vi "Playback Frame Crop Utility.vi"(8 "error in (no error)":errorcluster, 11 "Frame Grabber Data in":T2={"Camera Session"="", "Frame"=refnum, "AVI Refnum"=refnum, "Codecs"=[], "Frame number"=0, "Tracking File Refnum"=refnum, "Tick Count"=0, "Probe Object"=refnum, "Playback Probe Data"=[], "Rigid Body"={"Position"={"x (mm)"=0.0, "y (mm)"=0.0, "z (mm)"=0.0}, "Orientation"={"Pitch (rad)"=0.0, "Yaw (rad)"=0.0, "Roll (rad)"=0.0}, "Quaternion"={"qx"=0.0, "qy"=0.0, "qz"=0.0, "qw"=0.0}, "Tracked?"=FALSE}, "Total no frames playback"=0, "Video FPS"=0.0, "Camera connected?"=FALSE, "Scene"=refnum, "Cropped Frame"=refnum, "Tracker FPS"=0.0, "Crop ROI"=[], "Presentation Values"=[], "Elapsed time (ms)"=0, "Camera frames playback"=0, "Refnums"={"Live Refnum"=refnum, "Record Refnum"=refnum, "Playback Refnum"=refnum, "Frame Slider Refnum"=refnum, "Pause Refnum"=refnum, "Home Refnum"=refnum, "Set Crop Refnum"=refnum, "Clear Crop Refnum"=refnum, "stop refnum"=refnum, "Playback Rate Refnum"=refnum, "Presentation Refnum"=refnum, "Crop Time Frame Slider Refnum"=refnum, "Cancel Save Refnum"=refnum, "Reverse Playback Refnum"=refnum, "Recording Settings Refnum"=refnum, "Continuous Playback Refnum"=refnum, "Annotation Refnum"=refnum, "Export All Refnum"=refnum, "Export List Refnum"=refnum, "Fill List Refnum"=refnum, "Save Crop Refnum"=refnum, "Skip Forward Refnum"=refnum, "Skip Backward Refnum"=refnum, "Single Annotation Refnum"=refnum, "Load Refnum"=refnum, "Set Start Refnum"=refnum, "Set End Refnum"=refnum, "Add to List Refnum"=refnum, "List of Annotations Refnum"=refnum, "Camera Frame Refnum"=refnum}, "Dimensions"={"Probe Dimensions"={"Probe Width"=0.0, "Probe Depth"=1.0, "Probe Height"=0.0}, "Room Dimensions"={"Room Width"=0.0, "Room Depth"=0.0, "Room Height"=0.0}}, "Playback Data As Strings"=[], "Cropped Tracking File Refnum"=refnum, "Cropped AVI Refnum"=refnum, "Header"=[], "Total euclidian distance"=0.0, "Annotation File Path"=path "", "Playback File Path"=path "", "Size per frame"=0.0, "Ground Truth File Refnum"=refnum, "Annotation Array"=[], "Annotation TIFFs Folder"=path "", "overwriting open file?"=FALSE}) -> (0 "error out":errorcluster, 1 "Continue playback?":bool, 2 "Image":T1, 3 "Frame Grabber Data out":T2={"Camera Session"="", "Frame"=refnum, "AVI Refnum"=refnum, "Codecs"=[], "Frame number"=0, "Tracking File Refnum"=refnum, "Tick Count"=0, "Probe Object"=refnum, "Playback Probe Data"=[], "Rigid Body"={"Position"={"x (mm)"=0.0, "y (mm)"=0.0, "z (mm)"=0.0}, "Orientation"={"Pitch (rad)"=0.0, "Yaw (rad)"=0.0, "Roll (rad)"=0.0}, "Quaternion"={"qx"=0.0, "qy"=0.0, "qz"=0.0, "qw"=0.0}, "Tracked?"=FALSE}, "Total no frames playback"=0, "Video FPS"=0.0, "Camera connected?"=FALSE, "Scene"=refnum, "Cropped Frame"=refnum, "Tracker FPS"=0.0, "Crop ROI"=[], "Presentation Values"=[], "Elapsed time (ms)"=0, "Camera frames playback"=0, "Refnums"={"Live Refnum"=refnum, "Record Refnum"=refnum, "Playback Refnum"=refnum, "Frame Slider Refnum"=refnum, "Pause Refnum"=refnum, "Home Refnum"=refnum, "Set Crop Refnum"=refnum, "Clear Crop Refnum"=refnum, "stop refnum"=refnum, "Playback Rate Refnum"=refnum, "Presentation Refnum"=refnum, "Crop Time Frame Slider Refnum"=refnum, "Cancel Save Refnum"=refnum, "Reverse Playback Refnum"=refnum, "Recording Settings Refnum"=refnum, "Continuous Playback Refnum"=refnum, "Annotation Refnum"=refnum, "Export All Refnum"=refnum, "Export List Refnum"=refnum, "Fill List Refnum"=refnum, "Save Crop Refnum"=refnum, "Skip Forward Refnum"=refnum, "Skip Backward Refnum"=refnum, "Single Annotation Refnum"=refnum, "Load Refnum"=refnum, "Set Start Refnum"=refnum, "Set End Refnum"=refnum, "Add to List Refnum"=refnum, "List of Annotations Refnum"=refnum, "Camera Frame Refnum"=refnum}, "Dimensions"={"Probe Dimensions"={"Probe Width"=0.0, "Probe Depth"=1.0, "Probe Height"=0.0}, "Room Dimensions"={"Room Width"=0.0, "Room Depth"=0.0, "Room Height"=0.0}}, "Playback Data As Strings"=[], "Cropped Tracking File Refnum"=refnum, "Cropped AVI Refnum"=refnum, "Header"=[], "Total euclidian distance"=0.0, "Annotation File Path"=path "", "Playback File Path"=path "", "Size per frame"=0.0, "Ground Truth File Refnum"=refnum, "Annotation Array"=[], "Annotation TIFFs Folder"=path "", "overwriting open file?"=FALSE}, 4 "Time elapsed (s)":dbl, 5 "Camera frame number":i32)   [LabVIEW 2017]
uses:
  Controls/Frame Grabber Data.ctl
  <vilib>/userdefined/High Color/IMAQdx.ctl
  <vilib>/vision/Image Controls.llb/IMAQ Image.ctl
  <vilib>/vision/Avi.llb/IMAQ AVI2 Refnum.ctl
  Controls/Rigid Body Info.ctl
  Controls/Position.ctl
  Controls/Orientation.ctl
  Controls/Refnums.ctl
  Controls/Recording Settings.ctl
  Controls/Operator Settings.ctl
  Controls/Operator.ctl
  Controls/Patient Settings.ctl
  Controls/Dimensions.ctl
  Controls/Room Dimensions.ctl
  <vilib>/vision/NI_Vision_Development_Module.lvlib
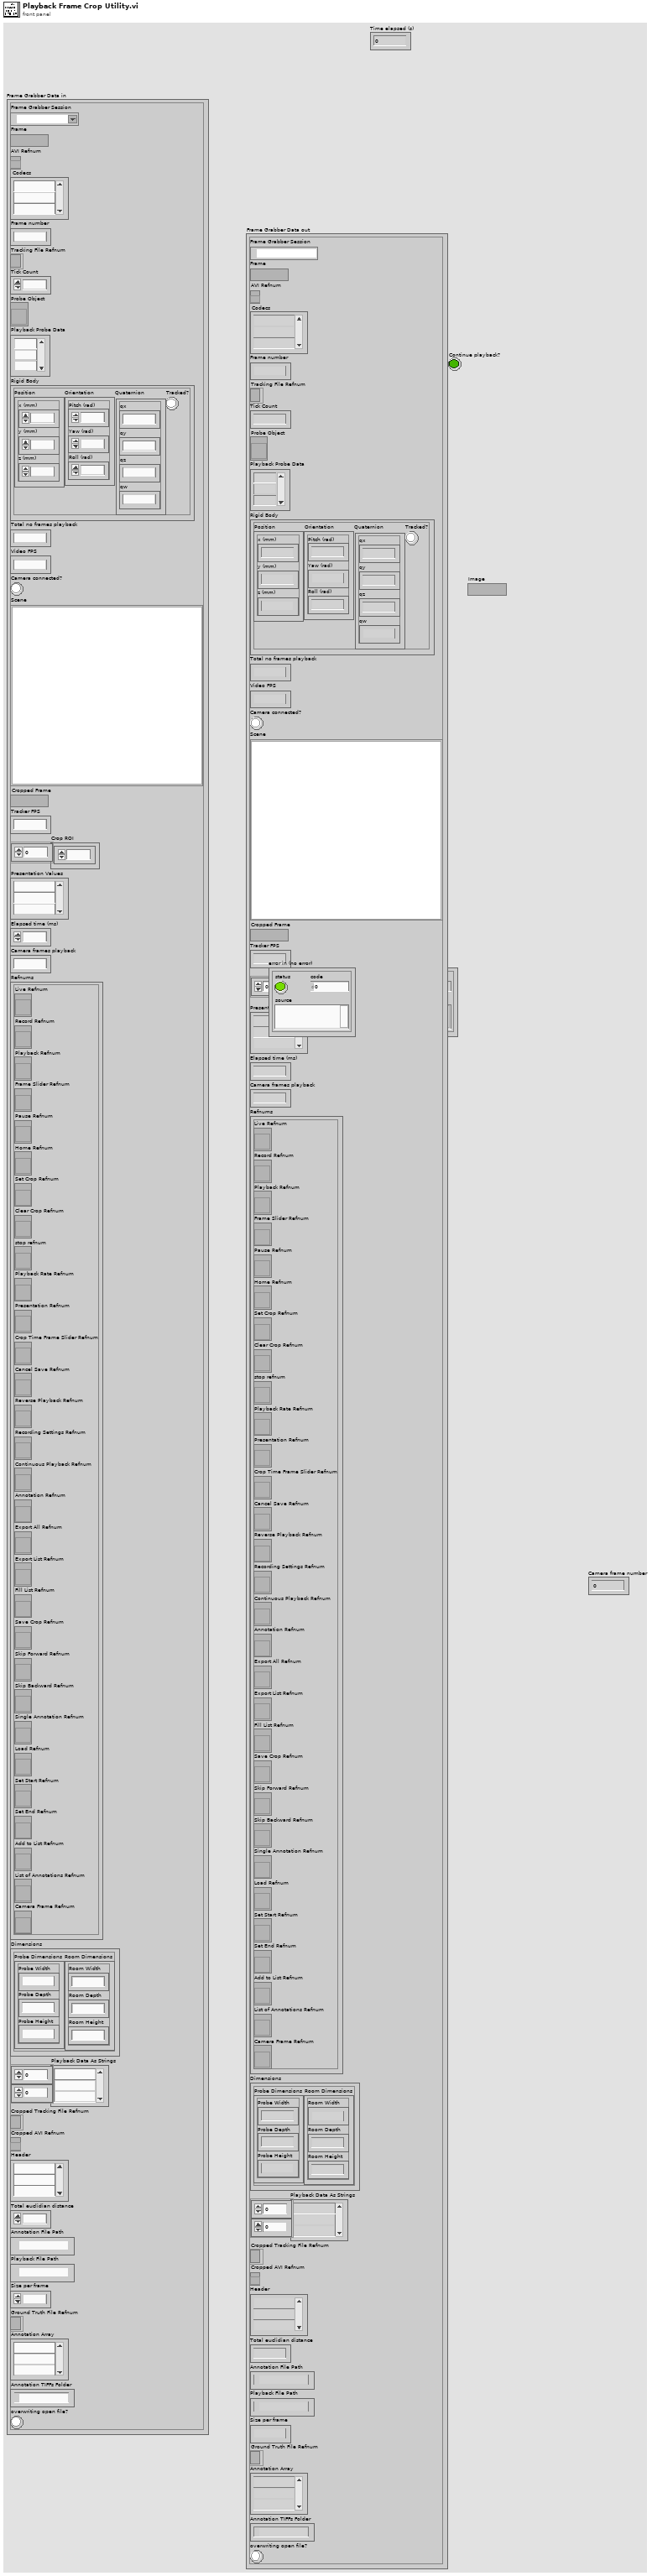
[diagram p1: front panel]
types:
  T1 = typedef "IMAQ Image.ctl" = refnum<image>
  T2 = typedef "Frame Grabber Data.ctl" = cluster{"Camera Session":T3, "Frame":T1, "AVI Refnum":T4, "Codecs":string[], "Frame number":u32, "Tracking File Refnum":refnum<file>, "Tick Count":u32, "Probe Object":refnum<vi>, "Playback Probe Data":dbl[][], "Rigid Body":T5, "Total no frames playback":i32, "Video FPS":dbl, "Camera connected?":bool, "Scene":refnum<vi>, "Cropped Frame":T1, "Tracker FPS":dbl, "Crop ROI":i32[], "Presentation Values":string[], "Elapsed time (ms)":u32, "Camera frames playback":u32, "Refnums":T8, "Dimensions":T9, "Playback Data As Strings":string[][], "Cropped Tracking File Refnum":refnum<file>, "Cropped AVI Refnum":T4, "Header":string[], "Total euclidian distance":dbl, "Annotation File Path":path, "Playback File Path":path, "Size per frame":dbl, "Ground Truth File Refnum":refnum<file>, "Annotation Array":string[], "Annotation TIFFs Folder":path, "overwriting open file?":bool}
  T3 = typedef "IMAQdx.ctl" = refnum<k21>
  T4 = typedef "IMAQ AVI2 Refnum.ctl" = refnum<k20>
  T5 = typedef "Rigid Body Info.ctl" = cluster{"Position":T6, "Orientation":T7, "Quaternion":cluster{"qx":sgl, "qy":sgl, "qz":sgl, "qw":sgl}, "Tracked?":bool}
  T6 = typedef "Position.ctl" = cluster{"x (mm)":sgl, "y (mm)":sgl, "z (mm)":sgl}
  T7 = typedef "Orientation.ctl" = cluster{"Pitch (rad)":sgl, "Yaw (rad)":sgl, "Roll (rad)":sgl}
  T8 = typedef "Refnums.ctl" = cluster{"Live Refnum":refnum<vi>, "Record Refnum":refnum<vi>, "Playback Refnum":refnum<vi>, "Frame Slider Refnum":refnum<vi>, "Pause Refnum":refnum<vi>, "Home Refnum":refnum<vi>, "Set Crop Refnum":refnum<vi>, "Clear Crop Refnum":refnum<vi>, "stop refnum":refnum<vi>, "Playback Rate Refnum":refnum<vi>, "Presentation Refnum":refnum<vi>, "Crop Time Frame Slider Refnum":refnum<vi>, "Cancel Save Refnum":refnum<vi>, "Reverse Playback Refnum":refnum<vi>, "Recording Settings Refnum":refnum<vi>, "Continuous Playback Refnum":refnum<vi>, "Annotation Refnum":refnum<vi>, "Export All Refnum":refnum<vi>, "Export List Refnum":refnum<vi>, "Fill List Refnum":refnum<vi>, "Save Crop Refnum":refnum<vi>, "Skip Forward Refnum":refnum<vi>, "Skip Backward Refnum":refnum<vi>, "Single Annotation Refnum":refnum<vi>, "Load Refnum":refnum<vi>, "Set Start Refnum":refnum<vi>, "Set End Refnum":refnum<vi>, "Add to List Refnum":refnum<vi>, "List of Annotations Refnum":refnum<vi>, "Camera Frame Refnum":refnum<vi>}
  T9 = typedef "Dimensions.ctl" = cluster{"Probe Dimensions":cluster{"Probe Width":sgl, "Probe Depth":sgl, "Probe Height":sgl}, "Room Dimensions":T10}
  T10 = typedef "Room Dimensions.ctl" = cluster{"Room Width":dbl, "Room Depth":dbl, "Room Height":dbl}
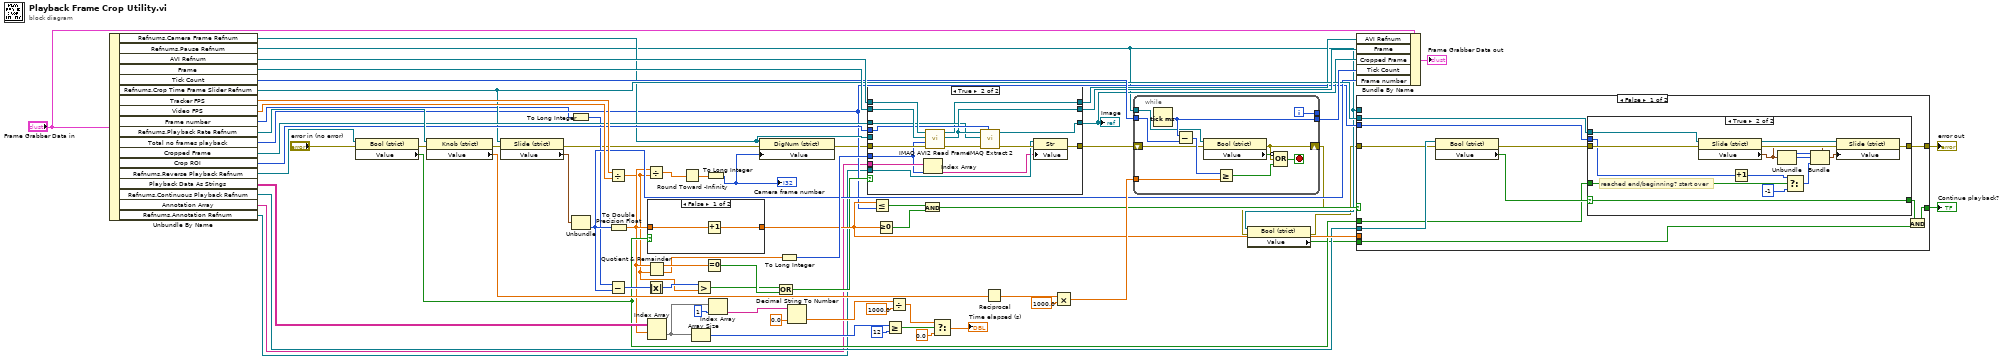
[diagram p0: block diagram]
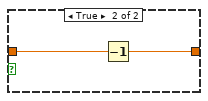
[diagram p2: hidden frame]
diagram:
  n1 = Unbundle By Name("Frame Grabber Data in") -> ("Refnums.Camera Frame Refnum"=w20:refnum<vi>, "Refnums.Pause Refnum"=w6:refnum<vi>, "AVI Refnum"=w71:T4, "Frame"=w72:T1, "Tick Count"=w65:u32, "Refnums.Crop Time Frame Slider Refnum"=w51:refnum<vi>, "Tracker FPS"=w64:dbl, "Video FPS"=w63:dbl, "Frame number"=w15:u32, "Refnums.Playback Rate Refnum"=w59:refnum<vi>, "Total no frames playback"=w18:i32, "Cropped Frame"=w54:T1, "Crop ROI"=w53:i32[], "Refnums.Reverse Playback Refnum"=w47:refnum<vi>, "Playback Data As Strings"=w43:string[][], "Refnums.Continuous Playback Refnum"=w19:refnum<vi>, "Annotation Array"=w8:string[], "Refnums.Annotation Refnum"=w7:refnum<vi>)
  n2 = property class="Bool (strict)"(reference=w47, error in="error in (no error)") -> (error out=w48:errorcluster, "Value"=w17:bool)  [unwired: 1 out]
  n3 = property class="Knob (strict)"(reference=w59, error in=w48) -> (error out=w60:errorcluster, "Value"=w61:dbl)  [unwired: 1 out]
  n4 = property class="Slide (strict)"(reference=w51, error in=w60) -> (error out=w13:errorcluster, "Value"=w57:cluster{i32, i32, i32})  [unwired: 1 out]
  n5 = To Long Integer(number=w15) -> (32bit integer=w24:i32)
  n6 = Unbundle(w57) -> (w25:i32)  [unwired: 2 out]
  n7 = Divide(x=w64, y=w63) -> (x/y=w10:dbl)
  n8 = Subtract(x=w24, y=w25) -> (x-y=w26:i32)
  n9 = To Double Precision Float(number=w25) -> (double precision float=w11:dbl)
  n10 = Divide(x=w11, y=w10) -> (x/y=w9:dbl)
  n11 = Absolute Value(x=w26) -> (abs(x)=w23:i32)
  n12 = case shown="False" w17 {
    tunnel: [w74 w75] -> w45
    tunnel: w11 -> [w73 w76]
    frame False {
      n13 = Increment(x=w73) -> (x+1=w74:dbl)
    }
    frame True {
      n14 = Decrement(x=w76) -> (x-1=w75:dbl)
    }
  }
  n15 = Quotient & Remainder(x=w11, y=w10) -> (x-y*floor(x/y)=w28:dbl, floor(x/y)=w14:dbl)
  n16 = Index Array(array=w43, index (row)=w11) -> (element=w39:string[])  [unwired: 1 in]
  n17 = Round Toward -Infinity(1:w9) -> (0:w2:dbl)
  n18 = Array Size(array=w39) -> (size(s)=w42:i32)
  n19 = Greater?(x=w23, y=w10) -> (0:w22:bool)
  n20 = Equal To 0?(x=w28) -> (x = 0?=w27:bool)
  n21 = To Long Integer(number=w2) -> (32bit integer=w1:i32)
  "Camera frame number" <- w1
  n22 = Index Array(array=w39, index=1) -> (element=w37:string)
  n23 = property class="DigNum (strict)"(reference=w20, error in=w13, "Value"=w1) -> (error out=w12:errorcluster)  [unwired: 1 out]
  n24 = Or(x=w22, y=w27) -> (x .or. y?=w21:bool)
  n25 = To Long Integer(number=w14) -> (32bit integer=w58:i32)
  n26 = Decimal String To Number(string=w37, default (0L)=0.0 ("default (0 I32)")) -> (number=w35:dbl)  [unwired: 1 in, 1 out]
  n27 = case shown="True" w21 {
    tunnel: [w78 w91] -> w30
    tunnel: w72 -> [w79 w95]
    tunnel: w71 -> [w77 w94]
    tunnel: [w80 w83] -> w62
    tunnel: w12 -> [w80 w93]
    tunnel: w58 -> [_ w85]
    tunnel: w54 -> [w78 w88]
    tunnel: w53 -> [_ w90]
    tunnel: [w79 w89] -> w52
    tunnel: [w77 w87] -> w44
    tunnel: w20 -> [_ _]
    tunnel: w8 -> [_ w86]
    tunnel: w7 -> [_ w82]
    frame False {
    }
    frame True {
      n28 = Index Array(array=w86, index=w85) -> (element=w81:string)
      n29 = call "IMAQ AVI2 Read Frame"("error in (no error)"=w93, "Frame Number"=w85, "Image"=w95, "AVI Refnum"=w94) -> ("error out"=w92:errorcluster, "Image Out"=w89:T1, "AVI Refnum (duplicate)"=w87:T4)  [unwired: 5 in]
      n30 = call "IMAQ Extract 2"("Optional Rectangle"=w90, "error in (no error)"=w92, "Image Dst"=w88, "Image Src"=w89) -> ("error out"=w84:errorcluster, "Image Dst Out"=w91:T1)  [unwired: 6 in]
      n31 = property class="Str"(reference=w82, error in=w84, "Value"=w81) -> (error out=w83:errorcluster)  [unwired: 1 out]
    }
  }
  "Image" <- w30
  n32 = Less Or Equal?(x=w45, y=w18) -> (x <= y?=w55:bool)
  n33 = Greater Or Equal To 0?(x=w45) -> (x >= 0?=w46:bool)
  n34 = Greater Or Equal?(x=w42, y=12) -> (x >= y?=w40:bool)
  n35 = Divide(x=w35, y=1000.0) -> (x/y=w33:dbl)
  n36 = And(x=w55, y=w46) -> (x .and. y?=w50:bool)
  n37 = Select(t=w33, s=w40, f=0.0) -> (s? t:f=→"Time elapsed (s)":dbl)
  n38 = Reciprocal(x=w61) -> (1/x=w68:dbl)
  n39 = Multiply(x=w68, y=1000.0) -> (x*y=w66:dbl)
  n40 = while {
    tunnel: [w106] -> w69
    tunnel: w66 -> [w104]
    tunnel: w65 -> [w103]
    shift-right: [w99] -> w5
    shift-left: w62 -> [w100]
    tunnel: w6 -> [w98]
    tunnel: [w96] -> _
    i -> [w96]
    stop <- w102 stop-if-true
    n41 = Tick Count (ms)() -> (millisecond timer value=w106:u32)
    n42 = Subtract(x=w106, y=w103) -> (x-y=w105:u32)
    n43 = property class="Bool (strict)"(reference=w98, error in=w100) -> (error out=w99:errorcluster, "Value"=w97:bool)  [unwired: 1 out]
    n44 = Greater Or Equal?(x=w105, y=w104) -> (x >= y?=w101:bool)
    n45 = Compound Arithmetic op=OR(invert w97, w99, w101) -> (w102:bool)
  }
  n46 = property class="Bool (strict)"(reference=w6, error in=w5) -> (error out=w4:errorcluster, "Value"=w3:bool)  [unwired: 1 out]
  n47 = Bundle By Name(cluster="Frame Grabber Data in", "AVI Refnum"=w44, "Frame"=w52, "Cropped Frame"=w30, "Tick Count"=w69, "Frame number"=w25) -> (→"Frame Grabber Data out":T2)
  n48 = case shown="False" w50 {
    tunnel: w4 -> [w114 w136]
    tunnel: w6 -> [_ _]
    tunnel: w45 -> [_ _]
    tunnel: w51 -> [w117 _]
    tunnel: [w116 w136] -> w29
    tunnel: w19 -> [w115 _]
    tunnel: w18 -> [w111 _]
    tunnel: w17 -> [w110 _]
    tunnel: [w108 w135] -> w16
    tunnel: w3 -> [w107 w135]
    frame False {
      n49 = property class="Bool (strict)"(reference=w115, error in=w114) -> (error out=w113:errorcluster, "Value"=w112:bool)  [unwired: 1 out]
      n50 = case shown="True" w112 {
        selector: w112 -> [w118 w122]
        tunnel: w117 -> [_ w134]
        tunnel: [w119 w133] -> w116
        tunnel: w113 -> [w119 w132]
        tunnel: w111 -> [_ w124]
        tunnel: w110 -> [_ w123]
        tunnel: [w118 w122] -> w109
        frame False {
        }
        frame True {
          # "reached end/beginning? start over"
          n51 = property class="Slide (strict)"(reference=w134, error in=w132) -> (reference out=w131:refnum<vi>, error out=w127:errorcluster, "Value"=w121:cluster{i32, i32, i32})
          n52 = Increment(x=w124) -> (x+1=w120:i32)
          n53 = Unbundle(w121) -> (w128:i32, w129:i32)  [unwired: 1 out]
          n54 = Select(t=w120, s=w123, f=-1) -> (s? t:f=w125:i32)
          n55 = Bundle(cluster=w121, w128, w129, w125) -> (w130:cluster{i32, i32, i32})
          n56 = property class="Slide (strict)"(reference=w131, error in=w127, "Value"=w130) -> (error out=w133:errorcluster)  [unwired: 1 out]
        }
      }
      n57 = And(x=w109, y=w107) -> (x .and. y?=w108:bool)
    }
    frame True {
    }
  }
  "error out" <- w29
  "Continue playback?" <- w16
